vi "Constructor.vi"(8 "error in":errorcluster, 10 "Comparison":string, 11 "Name":string) -> (0 "error out":errorcluster, 3 "StringMeasureLimit":refnum<class "StringMeasureLimit.lvclass">)   [LabVIEW 2021, in "ProligentXMLGenerator.lvlib" / "StringMeasureLimit.lvclass"]
uses:
  StringMeasureLimit.lvclass
  StringMeasureLimit.lvclass/StringMeasureLimit.ctl
  MeasureLimit/MeasureLimit.lvclass
  C:/Projects/proligent-xml-generator-labview/src/ProligentXMLGenerator/Measure/MeasureLimit/MeasureLimit.lvclass
  C:/Projects/proligent-xml-generator-labview/src/ProligentXMLGenerator/Measure/StringMeasureLimit/StringMeasureLimit.lvclass
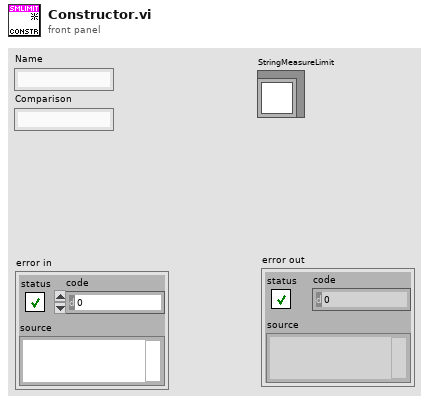
[diagram p1: front panel]
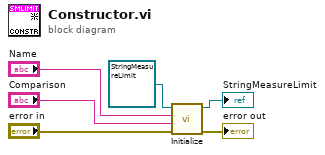
[diagram p0: block diagram]
diagram:
  n1 = call "Initialize.vi"("error in"="error in", "LimitExpression"="Comparison", "Name"="Name", "MeasureLimit in"=refnum<class "StringMeasureLimit.lvclass"> refnum ("ProligentResultProcessor:StringMeasureLimit")) -> ("error out"=→"error out":errorcluster, "MeasureLimit out"=→"StringMeasureLimit":refnum<class "StringMeasureLimit.lvclass">)  [unwired: 6 in]
